vi "SpreadsheetStorage.vi"() -> ()   [LabVIEW 2014]
doc: "This VI uses the wave-generator sub-VI from ch 3 as the source for the data to be writen to a tab-delimited .txt file. It will output data in two columns along with the appropriate headers (Time & Displacement)"
panel:
  in  "Waveform Parameters":T1 {"Shape" items=["Sine", "Cosine", "DC Level", "Square", "User-Defined"]}
  in  "Digitizing Parameters":T2
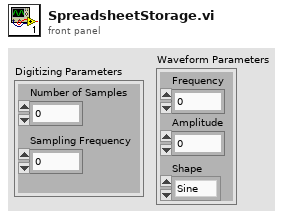
[diagram p1: front panel]
types:
  T1 = cluster{"Frequency ":dbl, "Amplitude ":dbl, "Shape":u16}
  T2 = cluster{"Number of Samples":dbl, "Sampling Frequency":dbl}
  T3 = enum16{"open", "replace", "create", "open or create", "replace or create", "replace or create with confirmation"}
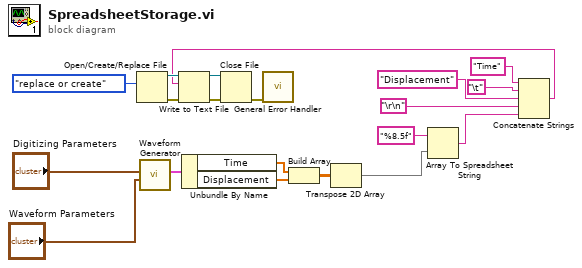
[diagram p0: block diagram]
diagram:
  n1 = Open/Create/Replace File(operation (0:open)=T3."replace or create") -> (refnum out=w20:refnum<file>, error out=w17:errorcluster)  [unwired: 5 in, 1 out]
  n2 = call "Waveform Generator.vi"("Waveform Parameters"="Waveform Parameters", "Digitizing Parameters"="Digitizing Parameters") -> ("Waveform Output"=w13:cluster{"Time":dbl[], "Displacement":dbl[]})  [unwired: 9 in]
  n3 = Unbundle By Name(w13) -> ("Time"=w12:dbl[], "Displacement"=w11:dbl[])
  n4 = Build Array(w12, w11) -> (w10:dbl[][])
  n5 = Transpose 2D Array(2D array=w10) -> (transposed array=w9:dbl[][])
  n6 = Array To Spreadsheet String(array=w9, 3:"%8.5f" ("format string")) -> (spreadsheet string=w3:string)  [unwired: 1 in]
  n7 = Concatenate Strings("Time" ("string"), "\t", "Displacement" ("string"), "\r\n", w3) -> (w2:string)
  n8 = Write to Text File(file (use dialog)=w20, text=w2, error in=w17) -> (refnum out=w19:refnum<file>, error out=w18:errorcluster)  [unwired: 1 in, 1 out]
  n9 = Close File(refnum=w19, error in=w18) -> (error out=w14:errorcluster)  [unwired: 1 out]
  n10 = call <vilib>:"General Error Handler.vi"("error in (no error)"=w14) -> ()  [unwired: 10 in, 5 out]
